vi "monochromatorCommandGetFilterLabel.vi"(8 "error in":errorcluster, 10 "filter_position":i32, 11 "monochromator":refnum<k24>) -> (0 "error out":errorcluster, 2 "label":string, 3 "monochromator":refnum<k24>)   [LabVIEW 2009]
doc: "Get filter label for a requested filter"
uses:
  C:/Users/anderson.chen/Desktop/Software Development/Cornerstone Series API (LV9)/Cornerstone DLL/Cornerstone.dll
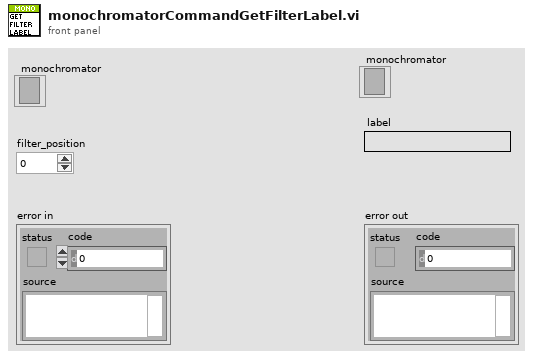
[diagram p1: front panel]
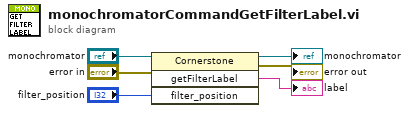
[diagram p0: block diagram]
diagram:
  n1 = invoke class="Cornerstone" method="getFilterLabel"(reference="monochromator", error in="error in", "filter_position"="filter_position") -> (reference out=→"monochromator":refnum<k24>, error out=→"error out":errorcluster, "getFilterLabel"=→"label":string)  [unwired: 1 in, 1 out]
